vi "MM9.InitLogDevs.vi"(0 "i ref in":refnum<vi>, 2 "InitObjs":string[](array[string]), 3 "ms timeout (10000)":i32=10000, 5 "error in (no error)":errorcluster) -> (14 "i ref out":refnum<vi>, 16 "InitObjs out":string[](array[string]), 17 "timed out":bool, 19 "error out":errorcluster)   [LabVIEW 2014, in "MM9.lvlib"]
doc: "Initializes log devices (whatever that is...)"
uses:
  MM9.lvlib
  CS_Core/CSSystem/CoreDefs/CoreDefs.call_type.ctl
  CS_Core/BaseProcess/BaseProcess.descriptor string definition.ctl
  CS_Core/CSSystem/CoreDefs/CoreDefs.rawDataType.ctl
  CS_Core/BaseProcess/BaseProcess.lvlib
  LEBITLib/LEBITLib.lvlib
panel:
  in  "CallClusterTyp":T1={"Object"="", "Selector"="", "CallType"=enum."synchronous", "Async Object"="", "Async Selector"="", "Data Descriptor"="", "Data"=[], "Error #"=0, "Expire"=0}
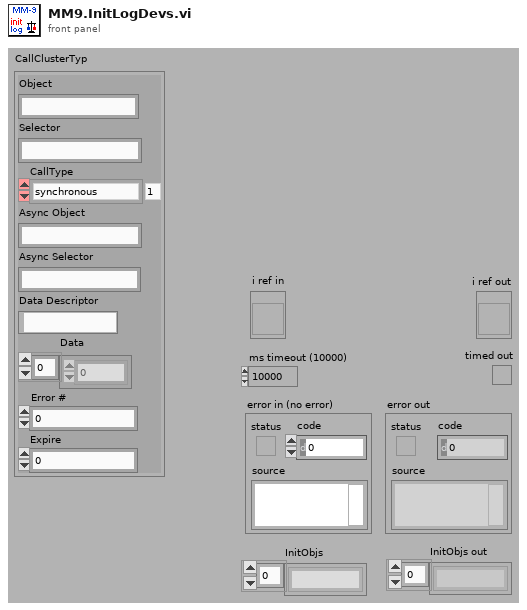
[diagram p1: front panel]
types:
  T1 = typedef "CoreDefs.call_type.ctl" = cluster{"Object":string, "Selector":string, "CallType":enum16{"simple", "synchronous", "asynchronous"}, "Async Object":string, "Async Selector":string, "Data Descriptor":T2, "Data":T3, "Error #":i32, "Expire":u32}
  T2 = typedef "BaseProcess.lvlib/BaseProcess.descriptor string definition.ctl" = string
  T3 = typedef "CoreDefs.rawDataType.ctl" = i8[]
  T4 = enum16{"simple", "synchronous", "asynchronous", "notification"}
  T5 = typedef "MM9.lvlib/MM9.i attribute.ctl" = cluster{"UsedObjs":string[], "ActScanStep":i32[], "AbortRequest":bool, "StopRequest":bool, "# cycles":i32, "Connected":bool, "MMStatus":T6, "# data":i32, "DIMServices":cluster{"MM6StatusString":string, "MM6StatusID":i32, "discArchiver":string, "discArchiverID":i32, "eventBuilder":string, "eventBuilderID":i32, "GUIIDString":string, "GUIIDStringID":i32}, "dataFile":string, "PGRunning":T7, "ConfigData":T8, "ExtraDataSets":T23}
  T6 = typedef "MM9.lvlib/MM9.status.ctl" = enum16{"loaded", "load_error", "config", "config_error", "init", "init_error", "data_reset", "data_reset_error", "running", "start_error", "run_error", "abort_requested", "aborted", "stop_requested", "stopped", "stop_error", "Connected", "NOTConnected"}
  T7 = typedef "PPG_ABC.lvlib/PPG_ABC.PG_Running.ctl" = i32
  T8 = typedef "LEBITDefs9.lvlib/LEBITDefs.ConfigData.ctl" = cluster{"GenConfig":T9, "Configs":T11[]}
  T9 = typedef "LEBITDefs9.lvlib/LEBITDefs.GenConfig.ctl" = cluster{"Mode":i32, "Logs":T10[]}
  T10 = typedef "LEBITDefs9.lvlib/LEBITDefs.Log.ctl" = cluster{"Name":string, "FctName":string, "Special":string}
  T11 = typedef "LEBITDefs9.lvlib/LEBITDefs.OneConfig.ctl" = cluster{"MCA":T12, "Timing":T13, "Scans":T16[], "FreqDevs":T17[], "CleanDev":T18, "NrCycles":i32, "Specials":T20[], "Delays":T21[], "DAC":T22}
  T12 = typedef "LEBITDefs9.lvlib/LEBITDefs.MCA.ctl" = cluster{"Name":string, "Address":string, "NrChannels":i32, "Gate":i32, "NrPipse":i32, "AcqDelay":i32}
  T13 = typedef "LEBITDefs9.lvlib/LEBITDefs.Timing.ctl" = cluster{"TimeTables":cluster{"TimeTable":T14}[], "Memories":T15[], "ScanX":string, "ScanY":string}
  T14 = typedef "LEBITDefs9.lvlib/LEBITDefs.Timetable.ctl" = dbl[]
  T15 = typedef "LEBITDefs9.lvlib/LEBITDefs.Memory.ctl" = cluster{"Device":string, "ExtTrig":bool, "TT2Use":i32, "PatternTable":string[]}
  T16 = typedef "LEBITDefs9.lvlib/LEBITDefs.ScanDev.ctl" = cluster{"Name":string, "FctName":string, "Values":dbl[], "NrScanVals":i32, "Special":string}
  T17 = typedef "LEBITDefs9.lvlib/LEBITDefs.FreqDev.ctl" = cluster{"Name":string, "Amp":dbl, "CenterFreq":dbl, "Time":dbl}
  T18 = typedef "LEBITDefs9.lvlib/LEBITDefs.CleanDev.ctl" = cluster{"Name":string, "CleanData":T19[]}
  T19 = typedef "LEBITDefs9.lvlib/LEBITDefs.CleanDataType.ctl" = cluster{"Amp":dbl, "Center":dbl, "Plus":dbl, "Minus":dbl, "Time":dbl}
  T20 = typedef "LEBITDefs9.lvlib/LEBITDefs.Special.ctl" = cluster{"Name":string, "FctName":string, "VerySpecial":string, "Data":dbl}
  T21 = typedef "LEBITDefs9.lvlib/LEBITDefs.Delay.ctl" = cluster{"Name":string, "Delay":dbl}
  T22 = typedef "LEBITDefs9.lvlib/LEBITDefs.DAC.ctl" = cluster{"Name":string, "Step1":i32, "Step2":i32}
  T23 = typedef "LEBITDefs9.lvlib/LEBITDefs.ExtraData.ctl" = cluster{"Ions":cluster{"ExcitIonMass":string, "ExcitIonCharge":i32, "CleanIons":cluster{"CleanIonMass":string, "CleanIonCharge":i32}[]}, "TimingDescription":cluster{"TimeTableDescription":cluster{"Times":string[]}[], "PatternTableDescription":cluster{"Pattern":string[]}[]}, "ScanUnits":string[]}[]
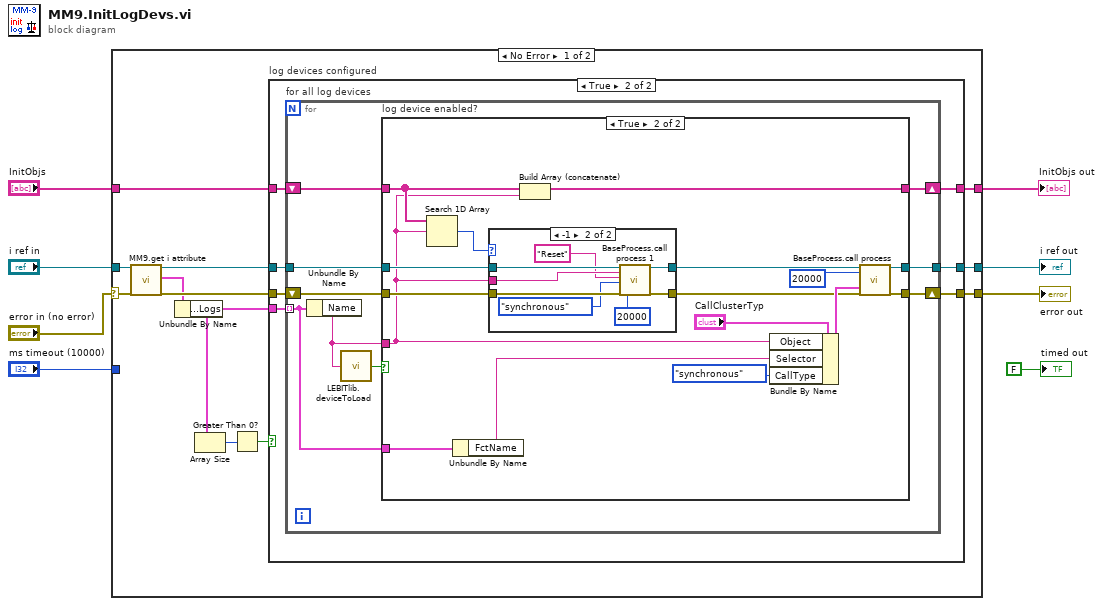
[diagram p0: block diagram]
diagram:
  n1 = case shown="No Error" "error in (no error)" {
    selector: "error in (no error)" -> [w11 w69]
    tunnel: "i ref in" -> [w16 w70]
    tunnel: [w15 w70] -> w7
    tunnel: [w14 w69] -> w6
    tunnel: "InitObjs" -> [w13 w71]
    tunnel: [w12 w71] -> w3
    tunnel: "ms timeout (10000)" -> [_ _]
    frame No Error {
      n2 = call "MM9.get i attribute.vi"("i ref in"=w16, "error in (no error)"=w11) -> ("i ref out"=w19:refnum<vi>, "i attribute"=w17:T5, "error out"=w18:errorcluster)  [unwired: 15 in]
      n3 = Unbundle By Name(w17) -> ("ConfigData.GenConfig.Logs"=w20:T10[])
      n4 = Array Size(array=w20) -> (size(s)=w9:i32)
      n5 = Greater Than 0?(x=w9) -> (x > 0?=w10:bool)
      n6 = case "log devices configured" shown="True" w10 {
        tunnel: w20 -> [_ w30]
        tunnel: w19 -> [w23 w29]
        tunnel: [w23 w28] -> w15
        tunnel: w18 -> [w22 w24]
        tunnel: [w22 w25] -> w14
        tunnel: w13 -> [w21 w27]
        tunnel: [w21 w26] -> w12
        frame False {
        }
        frame True {
          n7 = for "for all log devices" {
            tunnel: w30 -> [w37] mode=indexing
            tunnel: w29 -> [w39]
            tunnel: [w38] -> w28
            shift-right: [w36] -> w26
            shift-left: w27 -> [w35]
            shift-right: [w34] -> w25
            shift-left: w24 -> [w33]
            n8 = Unbundle By Name(w37) -> ("Name"=w31:string)
            n9 = call "LEBITlib.deviceToLoad.vi"("DeviceName"=w31) -> ("DeviceIsToLoad"=w32:bool)
            n10 = case "log device enabled?" shown="True" w32 {
              tunnel: w39 -> [w42 w51]
              tunnel: [w42 w54] -> w38
              tunnel: w33 -> [w41 w50]
              tunnel: w31 -> [_ w45]
              tunnel: [w41 w53] -> w34
              tunnel: w37 -> [_ w58]
              tunnel: w35 -> [w40 w46]
              tunnel: [w40 w44] -> w36
              frame False {
              }
              frame True {
                n11 = Search 1D Array(1D array=w46, element=w45) -> (index of element=w47:i32)  [unwired: 1 in]
                n12 = Unbundle By Name(w58) -> ("FctName"=w43:string)
                n13 = case shown="-1" w47 {
                  tunnel: w51 -> [w60 w68]
                  tunnel: w50 -> [w59 w67]
                  tunnel: [w60 w66] -> w49
                  tunnel: [w59 w65] -> w48
                  tunnel: w45 -> [_ w63]
                  frame 0, Default {
                  }
                  frame -1 {
                    n14 = call "BaseProcess.call process 1.vi"("i ref in"=w68, "Object"=w63, "Selector"="Reset", "CallType"=T4."synchronous", "error in (no error)"=w67, "timeout (ms)"=20000) -> ("i ref out"=w66:refnum<vi>, "error out"=w65:errorcluster)  [unwired: 11 in, 1 out]
                  }
                }
                n15 = Build Array (concatenate)(w46, w45) -> (w44:string[])
                n16 = Bundle By Name(cluster="CallClusterTyp", "Object"=w45, "Selector"=w43, "CallType"=enum16{"simple", "synchronous", "asynchronous"}."synchronous") -> (w57:T1)
                n17 = call "BaseProcess.call process.vi"("i ref in"=w49, "timeout (ms)"=20000, "call cluster in"=w57, "error in (no error)"=w48) -> ("i ref out"=w54:refnum<vi>, "error out"=w53:errorcluster)  [unwired: 13 in, 1 out]
              }
            }
          }
        }
      }
    }
    frame Error {
    }
  }
  "error out" <- w6
  "i ref out" <- w7
  "InitObjs out" <- w3
  "timed out" <- FALSE ("timed out")
